vi "AutoCorrelation Matrix (DBL).vi"(7 "initial?":bool, 9 "method":T1 items=["AutoCorrelation", "Pre-Windowed", "Post-Windowed", "Covariance", "Modified Covariance"], 10 "order":i32, 11 "X":dbl[](array[numeric])) -> (0 "error":i32, 3 "AutoCorrelation Matrix":T2)   [LabVIEW 2020, in "NI_AAL_SigProc.lvlib"]
doc: "Computes the autocorrelation matrix of the input sequence <B>X</B>. Wire data to the <B>X</B> input to determine the polymorphic instance to use or manually select the instance."
uses:
  <vilib>/Analysis/NI_AAL_SigProc.lvlib
  <vilib>/Analysis/Matrix/Datatypes/RealMatrix.ctl
  <vilib>/Analysis/2dsp.llb/AutoCorrelation Matrix Method.ctl
  <resource>/lvanlys.dll
  <vilib>/Analysis/Matrix/NI_Matrix.lvlib
panel:
  # "AutoCorrelation Matrix (DBL)"
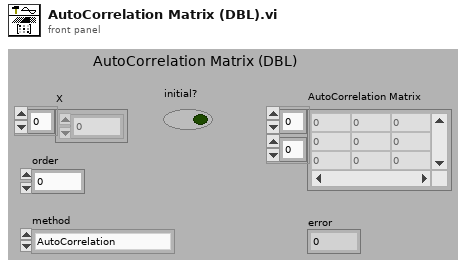
[diagram p1: front panel]
types:
  T1 = typedef "NI_AAL_SigProc.lvlib/AutoCorrelation Matrix Method.ctl" = i32
  T2 = typedef "NI_Matrix.lvlib/RealMatrix.ctl" = dbl[][]
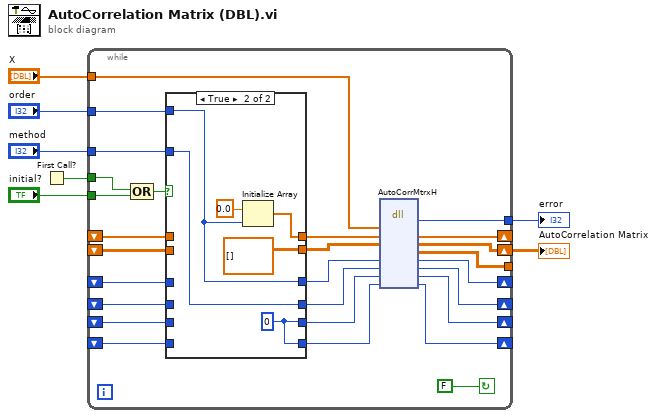
[diagram p0: block diagram]
diagram:
  n1 = First Call?() -> (First Call?: T/F=w1:bool)
  n2 = while {
    tunnel: "X" -> [w31]
    tunnel: "order" -> [w20]
    tunnel: "method" -> [w16]
    shift-right: [w30] -> w5
    shift-left: _ -> [w23]
    tunnel: [w29] -> w4
    shift-right: [w28] -> _
    shift-left: _ -> [w25]
    tunnel: "initial?" -> [w27]
    tunnel: [w21] -> _
    shift-right: [w18] -> _
    shift-left: _ -> [w17]
    shift-right: [w10] -> _
    shift-left: _ -> [w15]
    shift-right: [w9] -> _
    shift-left: _ -> [w14]
    shift-right: [w12] -> _
    shift-left: _ -> [w11]
    tunnel: w1 -> [w8]
    stop <- FALSE continue-if-true
    n3 = Compound Arithmetic op=OR(w8, w27) -> (w26:bool)
    n4 = case shown="True" w26 {
      tunnel: w25 -> [w37 _]
      tunnel: [w37 w43] -> w24
      tunnel: w23 -> [w36 _]
      tunnel: [w36 dbl[][] [] ("AutoCorrMtrx")] -> w22
      tunnel: w20 -> [_ w40]
      tunnel: [w38 w39] -> w19
      tunnel: w17 -> [w38 _]
      tunnel: w16 -> [_ w41]
      tunnel: [w35 w41] -> w10
      tunnel: w15 -> [w35 _]
      tunnel: [w34 w40] -> w9
      tunnel: w14 -> [w34 _]
      tunnel: [w33 w39] -> w13
      tunnel: w11 -> [w33 _]
      frame False {
      }
      frame True {
        w39 = 0 ("order")
        n5 = Initialize Array(0.0 ("element"), w40) -> (w43:dbl[])
      }
    }
    n6 = dll-call lib="e:/builds/penguin/labview/branches/2020/dev/dist/resource/lvanlys.*" fn="AutoCorrMtrxH"("X"=w31, "History"=w24, "AutoCorrMtrx"=w22, "order"=w9, "method"=w10, "index"=w19, "PrevSize"=w13) -> ("error"=w29:i32, "History"=w28:dbl[], "AutoCorrMtrx"=w30:dbl[][], "Matrix_X"=w21:dbl[][], "index"=w18:i32, "PrevSize"=w12:i32)  [unwired: 6 in, 3 out]
  }
  "AutoCorrelation Matrix" <- w5
  "error" <- w4
